vi "NI VeriStand - Search for All Items by GUID.vi"(8 "error in (no error)":errorcluster, 9 "Find All? (T)":bool=TRUE, 10 "Item GUID":string, 11 "Section Ref in":T1 format="%.0x") -> (0 "error out":errorcluster, 2 "Item Refs":T1[](array[typedef]) format="%.0x", 3 "Section Ref out":T1 format="%.0x", 4 "Found":bool)   [LabVIEW 2020, in "Custom Device Offline API.lvlib"]
uses:
  <vilib>/NI VeriStand/Custom Device Offline API/Custom Device Offline API.lvlib
  <vilib>/NI VeriStand/Custom Device API/Custom Device Item Ref.ctl
  NationalInstruments.VeriStand.SystemDefinitionAPI
  NationalInstruments.VeriStand.SystemStorage
  <vilib>/NI VeriStand/Custom Device API/Custom Device API.lvlib
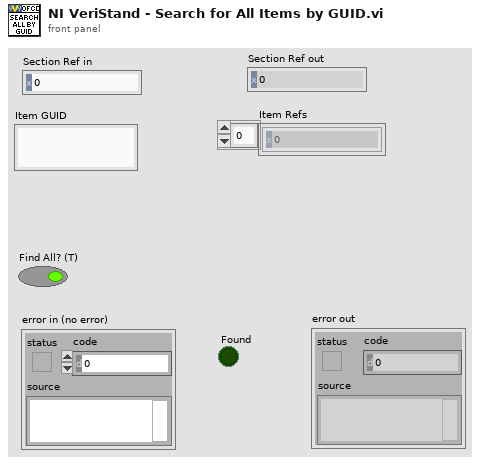
[diagram p1: front panel]
types:
  T1 = typedef "Custom Device API.lvlib/Custom Device Item Ref.ctl" = u64
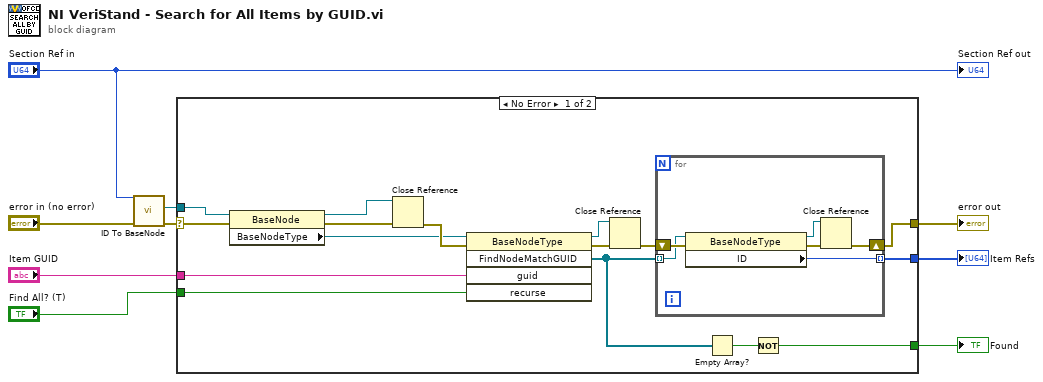
[diagram p0: block diagram]
diagram:
  n1 = call <vilib>:"ID To BaseNode.vi"("error in (no error)"="error in (no error)", "ID in"="Section Ref in") -> ("error out"=w9:errorcluster, "BaseNode"=w8:refnum<k24>)  [unwired: 7 in, 1 out]
  n2 = case shown="No Error" w9 {
    selector: w9 -> [w23 w32]
    tunnel: w8 -> [w24 _]
    tunnel: [w10 w32] -> w5
    tunnel: "Item GUID" -> [w17 _]
    tunnel: "Find All? (T)" -> [w16 _]
    tunnel: [w14 _] -> w2
    tunnel: [w11 _] -> w1
    frame No Error {
      n3 = property class="BaseNode"(reference=w24, error in=w23) -> (reference out=w21:refnum<k24>, error out=w22:errorcluster, "BaseNodeType"=w20:refnum<k24>)
      n4 = Close Reference(reference=w21, error in (no error)=w22) -> (error out=w25:errorcluster)
      n5 = invoke class="BaseNodeType" method="FindNodeMatchGUID"(reference=w20, error in=w25, "guid"=w17, "recurse"=w16) -> (reference out=w19:refnum<k24>, error out=w18:errorcluster, "FindNodeMatchGUID"=w12:refnum<k24>[])  [unwired: 1 in, 2 out]
      n6 = Close Reference(reference=w19, error in (no error)=w18) -> (error out=w13:errorcluster)
      n7 = for {
        shift-right: [w27] -> w10
        shift-left: w13 -> [w31]
        tunnel: w12 -> [w30] mode=indexing
        tunnel: [w26] -> w11 mode=indexing
        n8 = property class="BaseNodeType"(reference=w30, error in=w31) -> (reference out=w28:refnum<k24>, error out=w29:errorcluster, "ID"=w26:u64)
        n9 = Close Reference(reference=w28, error in (no error)=w29) -> (error out=w27:errorcluster)
      }
      n10 = Empty Array?(array=w12) -> (empty?=w15:bool)
      n11 = Not(x=w15) -> (.not. x?=w14:bool)
    }
    frame Error {
    }
  }
  "error out" <- w5
  "Found" <- w2
  "Item Refs" <- w1
  "Section Ref out" <- "Section Ref in"
